vi "Autonomous Independent sensor.vi"() -> ()   [LabVIEW 2013]
doc: "This VI is called when autonomous begins, and will automatically be terminated when autonomous ends. You can carry out timed or sensor driven robot movement independently without needing to return to the caller."
uses:
  Robot Global Data.vi
  <vilib>/Rock Robotics/WPI/Joystick/WPI_JoystickGetSetRefNum.vi
  <vilib>/Rock Robotics/WPI/RobotDrive/WPI_RobotDriveGetSetRefNum.vi
  <vilib>/Rock Robotics/WPI/RobotDrive/WPI_RobotDriveArcadeDrive_Standard(NoSaturation).vi
panel:
  out "Auton Switch On?":bool
  out "Numeric 4":i32
  out "Numeric 3":i32
  out "Numeric 2":i32
  out "Numeric":i32
  out "distance (mm) 2":dbl
  out "Angle 2":dbl
  out "distance (mm)":dbl
  out "Current Movement, for debugging":T1 {"Y Joystick Value" scale=1.0..-1.0; "X Joystick Value" scale=-1.0..1.0}
  in  "Array of robot movements":T2(array[cluster]) {"Y Joystick Value" scale=1.0..-1.0; "X Joystick Value" scale=-1.0..1.0}
  # "Be sure to right-click and choose Data Operations>>Make Current Value default if you want to save the array values with the VI"
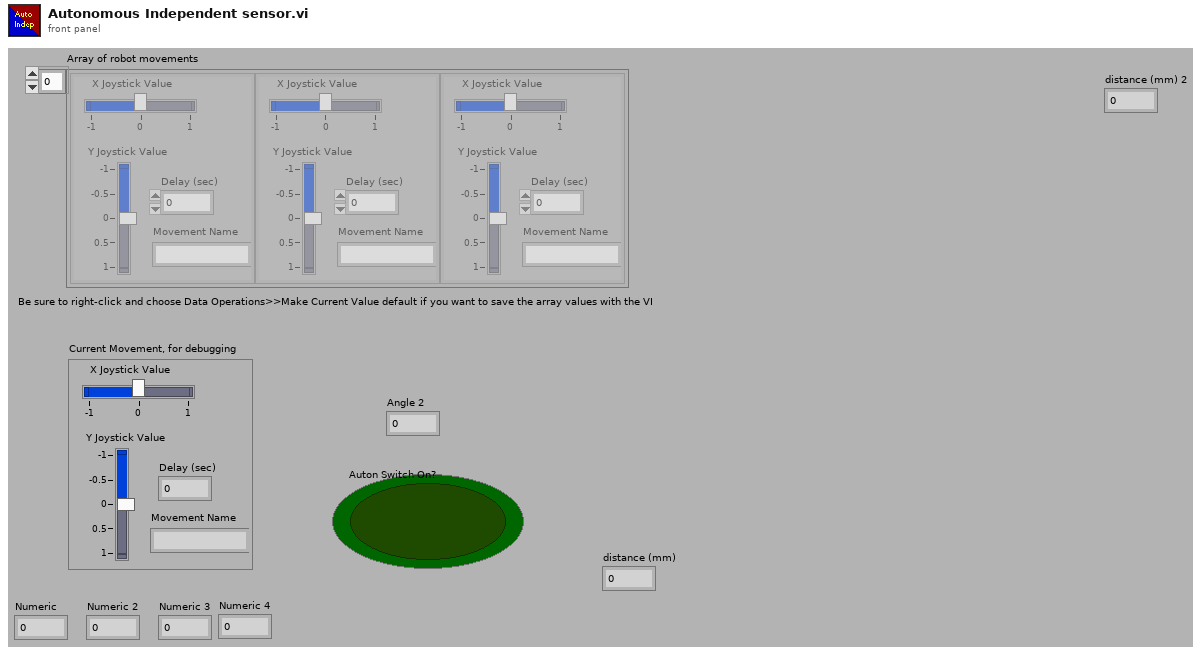
[diagram p1: front panel]
types:
  T1 = cluster{"X Joystick Value":dbl, "Y Joystick Value":dbl, "Delay (sec)":dbl, "Movement Name":string}
  T2 = cluster{"X Joystick Value":dbl, "Y Joystick Value":dbl, "Delay (sec)":dbl, "Movement Name":string}[]
  T3 = typedef "WPI_DigitalInputDevRef.ctl" = cluster{"DevStatus":errorcluster, "DIO Channel":T4, "Digital Module":T5}
  T4 = typedef "FPGA_DIOChannel.ctl" = enum8{"DIO 1", "DIO 2", "DIO 3", "DIO 4", "DIO 5", "DIO 6", "DIO 7", "DIO 8", "DIO 9", "DIO 10", "DIO 11", "DIO 12", "DIO 13", "DIO 14", "Invalid"}
  T5 = typedef "FPGA_TypedefDigitalModule.ctl" = enum16{"Digital Module 1", "Digital Module 2"}
  T6 = typedef "WPI_RobotDriveDevRef.ctl" = cluster{"DevStatus":errorcluster, "Motors[]":T7[], "Square Inputs":bool, "Max Output":dbl, "Isochronous":bool}
  T7 = typedef "WPI_MotorControlDeviceRef.ctl" = cluster{"DeviceStatus":errorcluster, "Type":enum16{"PWM", "CAN"}, "PWM":cluster{"Digital Module":T5, "PWM Channel":T8, "DeadBand":T9}, "CAN":cluster{"Device Number":u8, "Control Mode":T10, "Semaphore":T11, "Max Vout":dbl}, "Invert":bool, "TransformRef":T12, "InvTransformRef":T12}
  T8 = typedef "FPGA_DIOPWMChannel.ctl" = enum8{"PWM 1", "PWM 2", "PWM 3", "PWM 4", "PWM 5", "PWM 6", "PWM 7", "PWM 8", "PWM 9", "PWM 10", "Invalid"}
  T9 = typedef "WPI_PWMDeadband.ctl" = cluster{"Name":string, "maxPositivePwm":i32, "minPositivePwm":i32, "centerPwm":i32, "maxNegativePwm":i32, "minNegativePwm":i32, "angularRange":u16}
  T10 = typedef "WPI_CANJaguar_ControlMode.ctl" = enum8{"Percent VBus", "Current", "Speed", "Position", "Voltage"}
  T11 = typedef "Semaphore RefNum" = refnum<k1>
  T12 = typedef "WPI_PWMTransform_ConPane.ctl" = refnum<vi>
  T13 = typedef "WPI_GyroDevRef.ctl" = cluster{"DevStatus":errorcluster, "Analog Module":T14, "Analog Channel":T15, "Offset":dbl, "Gain (VoltsPerDegree/Second)":dbl}
  T14 = typedef "FPGA_TypedefAnalogModule.ctl" = enum16{"Analog Module 1", "Analog Module 2"}
  T15 = typedef "FPGA_AIChannel.ctl" = enum8{"AI 1", "AI 2", "AI 3", "AI 4", "AI 5", "AI 6", "AI 7", "AI 8", "Invalid"}
  T16 = typedef "WPI_AnalogChannelDevRef.ctl" = cluster{"DevStatus":errorcluster, "Analog Module":T14, "Analog Channel":T15}
  T17 = typedef "WPI_JoystickDevRef.ctl" = cluster{"Device":T18}
  T18 = typedef "WPI_JoystickDeviceEnum.ctl" = enum16{"USB 1", "USB 2", "USB 3", "USB 4", "Kinect 1", "Kinect 2"}
  T19 = cluster{"axis 1 (x)":dbl, "axis 2 (y)":dbl, "axis 3 (throttle)":dbl, "axis 4":dbl, "axis 5":dbl, "axis 6":dbl}
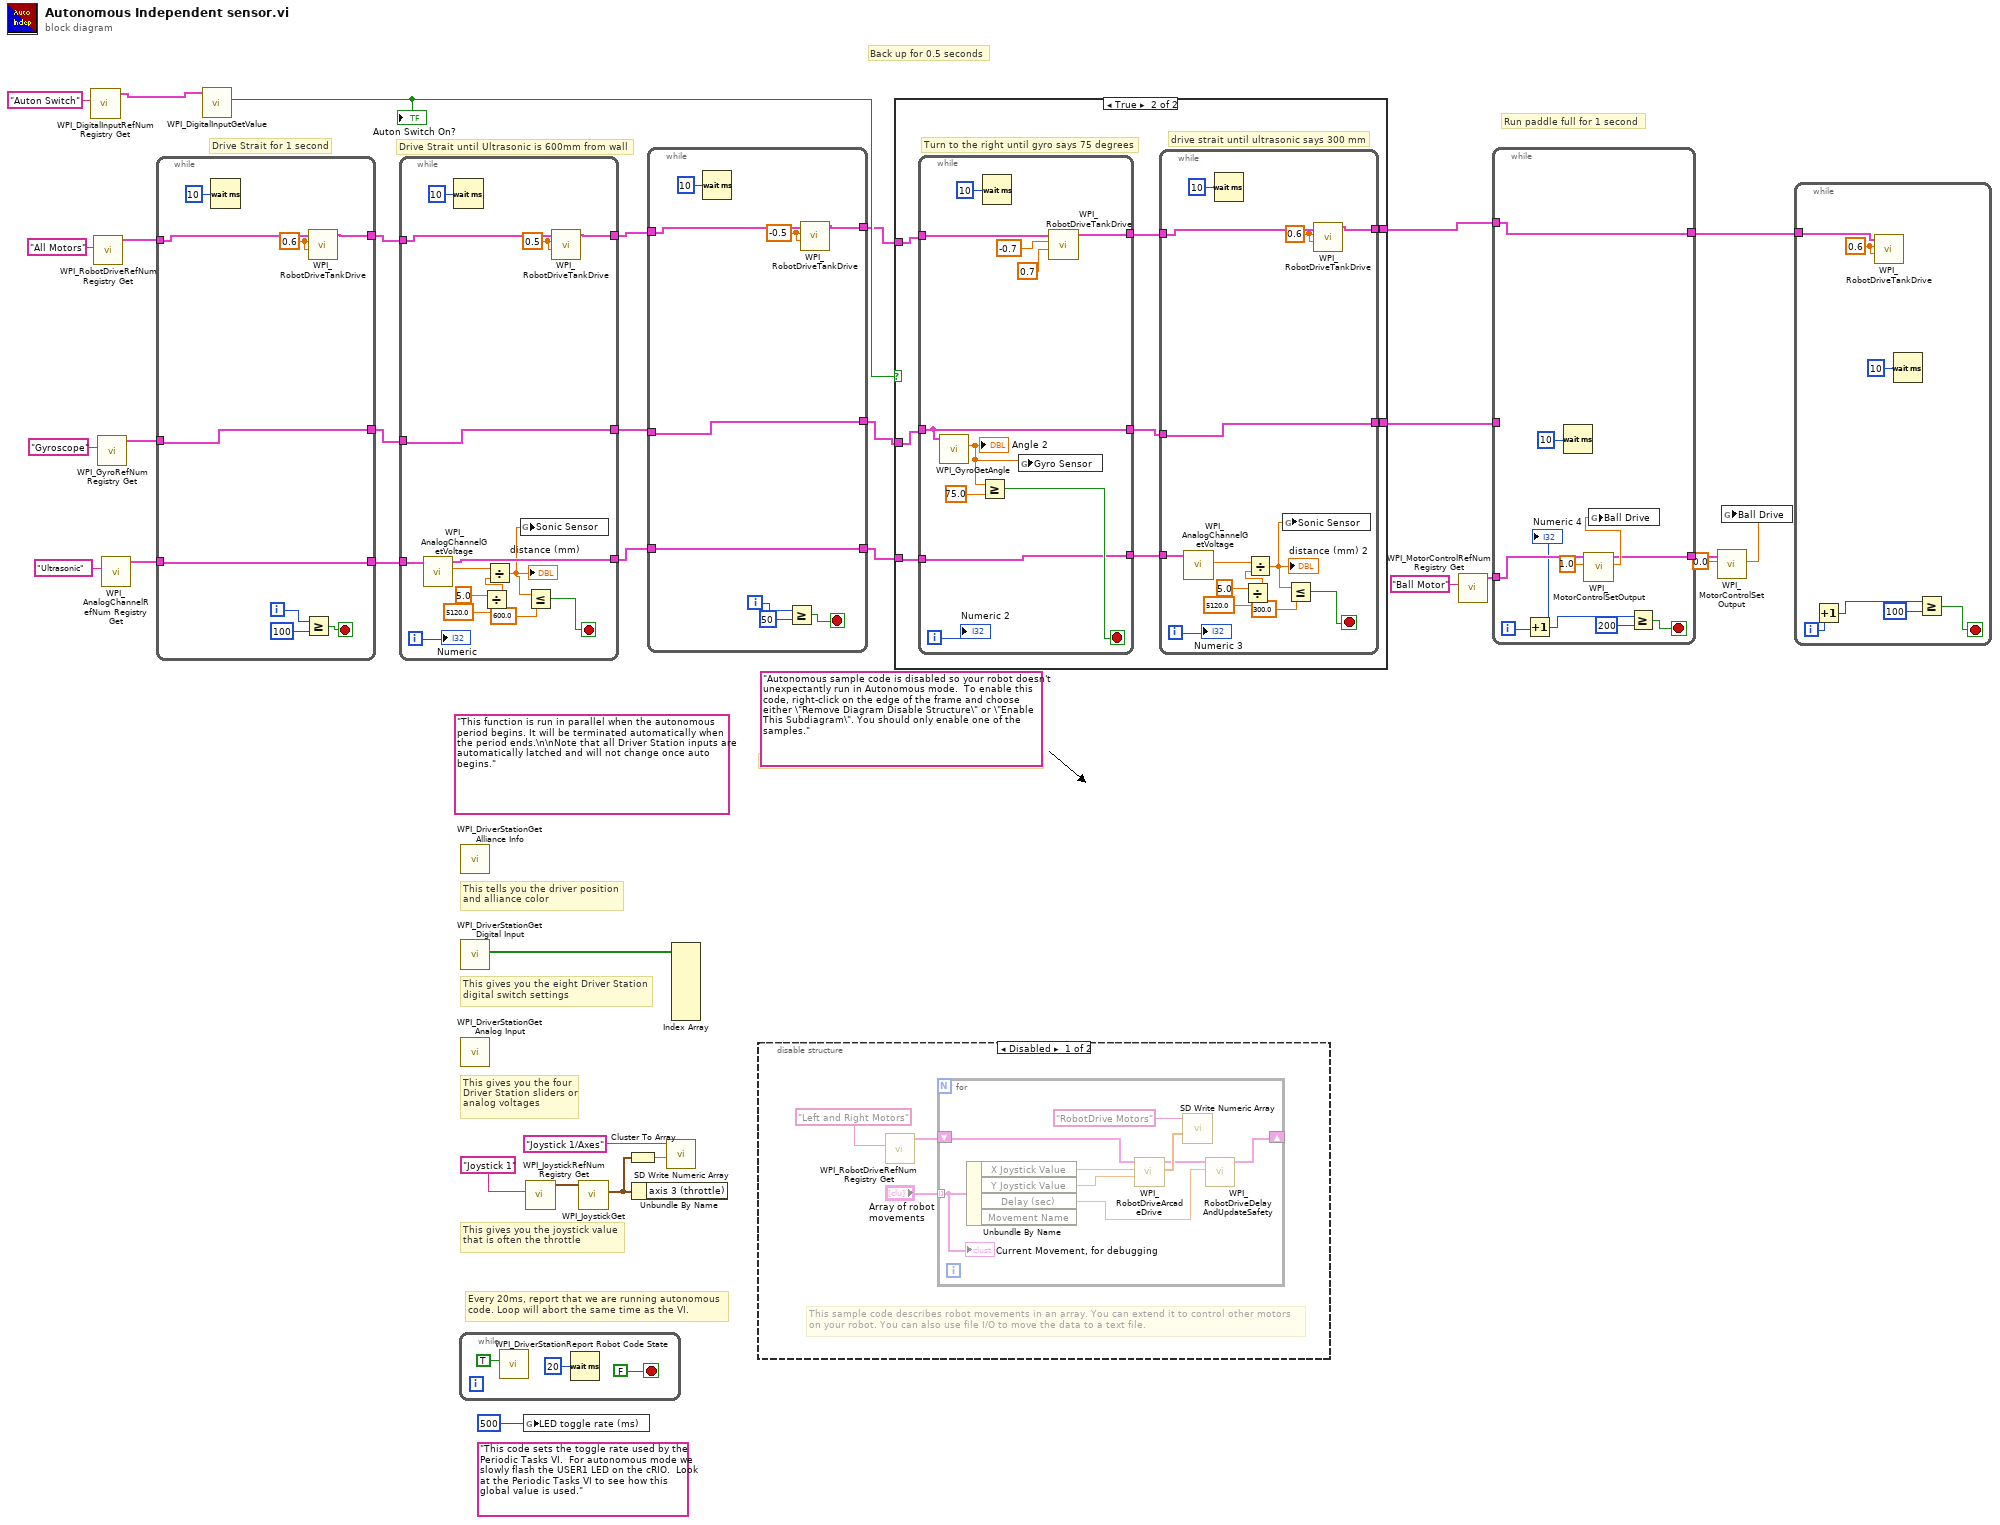
[diagram p0: block diagram]
diagram:
  (unwired) "This code sets the toggle rate used by the Periodic Tasks VI.  For autonomous mode we slowly flash the USER1 LED on the cRIO.  Look at the Periodic Tasks VI to see how this global value is used."
  (unwired) "Autonomous sample code is disabled so your robot doesn't unexpectantly run in Autonomous mode.  To enable this code, right-click on the edge of the frame and choose either \"Remove Diagram Disable Structure\" or \"Enable This Subdiagram\". You should only enable one of the samples."
  (unwired) "This function is run in parallel when the autonomous period begins. It will be terminated automatically when the period ends.\n\nNote that all Driver Station inputs are automatically latched and will not change once auto begins."
  # "Back up for 0.5 seconds"
  # "Run paddle full for 1 second"
  # "Drive Strait until Ultrasonic is 600mm from wall"
  # "Drive Strait for 1 second"
  # "Every 20ms, report that we are running autonomous\ncode. Loop will abort the same time as the VI."
  # "This gives you the joystick value\nthat is often the throttle"
  # "Use time and/or sensors to control how the robot drives."
  # "This tells you the driver position\nand alliance color"
  # "This gives you the eight Driver Station\ndigital switch settings"
  # "This gives you the four\nDriver Station sliders or\nanalog voltages"
  n1 = call <vilib>:"WPI_DigitalInputRefNum Registry Get.vi"("refnum name"="Auton Switch") -> ("DigitalInputDevRef"=w10:T3)  [unwired: 9 in, 1 out]
  n2 = call <vilib>:"WPI_RobotDriveRefNum Registry Get.vi"("refnum name"="All Motors") -> ("RobotDriveDevRef"=w16:T6)  [unwired: 9 in, 1 out]
  n3 = call <vilib>:"WPI_GyroRefNum Registry Get.vi"("refnum name"="Gyroscope") -> ("GyroDevRef"=w13:T13)  [unwired: 9 in, 1 out]
  n4 = call <vilib>:"WPI_AnalogChannelRefNum Registry Get.vi"("refnum name"="Ultrasonic") -> ("AIDeviceRef"=w17:T16)  [unwired: 9 in, 1 out]
  n5 = while {
    tunnel: w16 -> [w40]
    tunnel: w13 -> [w41]
    tunnel: [w39] -> w15
    tunnel: w17 -> [w37]
    tunnel: [w41] -> w12
    tunnel: [w37] -> w14
    i -> [w34]
    stop <- w35 stop-if-true
    w38 = 0.6 ("Left axis value")
    n6 = Wait (ms)(milliseconds to wait=u32 10) -> ()  [unwired: 1 out]
    n7 = Greater Or Equal?(x=w34, y=100) -> (x >= y?=w35:bool)
    n8 = call <vilib>:"WPI_RobotDriveTankDrive.vi"("Right axis value"=w38, "Left axis value"=w38, "RobotDriveDevRef"=w40) -> ("RobotDriveDevRef"=w39:T6)  [unwired: 6 in, 2 out]
  }
  n9 = call <vilib>:"WPI_DigitalInputGetValue.vi"("DigitalInputDevRef"=w10) -> ("Value"=w8:bool)  [unwired: 8 in, 2 out]
  "Auton Switch On?" <- w8
  n10 = while {
    tunnel: w15 -> [w45]
    tunnel: w12 -> [w46]
    tunnel: [w44] -> w7
    tunnel: w14 -> [w52]
    tunnel: [w46] -> w6
    tunnel: [w49] -> w5
    i -> [w47]
    stop <- w50 stop-if-true
    w43 = 0.5 ("Left axis value")
    n11 = call <vilib>:"WPI_AnalogChannelGetVoltage.vi"("AIDeviceRef"=w52) -> ("Voltage"=w55:dbl, "AIDeviceRef"=w49:T16)  [unwired: 8 in, 1 out]
    n12 = Wait (ms)(milliseconds to wait=u32 10) -> ()  [unwired: 1 out]
    n13 = Divide(x=5.0, y=5120.0) -> (x/y=w56:dbl)
    n14 = Divide(x=w55, y=w56) -> (x/y=w48:dbl)
    "distance (mm)" <- w48
    n15 = global write "Robot Global Data.vi" "Sonic Sensor"(w48) -> ()
    n16 = Less Or Equal?(x=w48, y=600.0) -> (x <= y?=w50:bool)
    n17 = call <vilib>:"WPI_RobotDriveTankDrive.vi"("Right axis value"=w43, "Left axis value"=w43, "RobotDriveDevRef"=w45) -> ("RobotDriveDevRef"=w44:T6)  [unwired: 6 in, 2 out]
    "Numeric" <- w47
  }
  n18 = while {
    stop <- FALSE stop-if-true
    n19 = call <vilib>:"WPI_DriverStationReport Robot Code State.vi"("Autonomous"=TRUE) -> ()  [unwired: 10 in, 1 out]
    n20 = Wait (ms)(milliseconds to wait=u32 20) -> ()  [unwired: 1 out]
  }
  n21 = call <vilib>:"WPI_DriverStationGet Alliance Info.vi"() -> ()  [unwired: 12 out]
  n22 = call <vilib>:"WPI_DriverStationGet Digital Input.vi"() -> ("Driver Station Digital Input (1-8)"=w33:bool[])  [unwired: 11 out]
  n23 = call <vilib>:"WPI_DriverStationGet Analog Input.vi"() -> ()  [unwired: 12 out]
  n24 = global write "Robot Global Data.vi" "LED toggle rate (ms)"(u32 500 ("LED ms toggle rate")) -> ()
  n25 = call <vilib>:"WPI_JoystickRefNum Registry Get.vi"("refnum name"="Joystick 1") -> ("JoystickDevRef"=w31:T17)  [unwired: 1 in, 9 out]
  n26 = call <vilib>:"WPI_JoystickGet.vi"("JoystickDevRef"=w31) -> ("Axes"=w28:T19)  [unwired: 1 in, 5 out]
  n27 = Cluster To Array(cluster=w28) -> (array=w29:dbl[])
  n28 = Unbundle By Name(w28) -> ()  [unwired: 1 out]
  n29 = while {
    tunnel: w7 -> [w67]
    tunnel: w6 -> [w68]
    tunnel: [w66] -> w4
    tunnel: [w68] -> w3
    tunnel: w5 -> [w64]
    tunnel: [w64] -> w2
    i -> [w63]
    stop <- w61 stop-if-true
    w65 = -0.5 ("Left axis value")
    n30 = Wait (ms)(milliseconds to wait=u32 10) -> ()  [unwired: 1 out]
    n31 = Greater Or Equal?(x=w63, y=50) -> (x >= y?=w61:bool)
    n32 = call <vilib>:"WPI_RobotDriveTankDrive.vi"("Right axis value"=w65, "Left axis value"=w65, "RobotDriveDevRef"=w67) -> ("RobotDriveDevRef"=w66:T6)  [unwired: 6 in, 2 out]
  }
  n33 = call <vilib>:"SD Write Numeric Array.vi"("Numeric Array"=w29, "Name"="Joystick 1/Axes") -> ()  [unwired: 8 in, 2 out]
  n34 = Index Array(array=w33) -> ()  [unwired: 8 in, 8 out]
  n35 = disable-structure shown="Disabled" {
    frame Disabled {
      # "This sample code describes robot movements in an array. You can extend it to control other motors\non your robot. You can also use file I/O to move the data to a text file."
      n36 = call <vilib>:"WPI_RobotDriveRefNum Registry Get.vi"("refnum name"="Left and Right Motors") -> ("RobotDriveDevRef"=w71:T6)  [unwired: 1 in, 9 out]
      n37 = for {
        shift-right: [w77] -> _
        shift-left: w71 -> [w78]
        tunnel: "Array of robot movements" -> [w73] mode=indexing
        n38 = Unbundle By Name(w73) -> ("X Joystick Value"=w76:dbl, "Y Joystick Value"=w75:dbl, "Delay (sec)"=w74:dbl)  [unwired: 1 out]
        n39 = call-poly <vilib>:"WPI_RobotDriveArcadeDrive.vi"("Y axis value"=w75, "X axis value"=w76, "RobotDriveDevRef"=w78) -> ("Motor Values"=w80:dbl[], "RobotDriveDevRef"=w79:T6)  [unwired: 1 in, 6 out]
        n40 = call <vilib>:"SD Write Numeric Array.vi"("Numeric Array"=w80, "Name"="RobotDrive Motors") -> ()  [unwired: 8 in, 2 out]
        n41 = call <vilib>:"WPI_RobotDriveDelayAndUpdateSafety.vi"("Delay (s)"=w74, "RobotDriveDevRef"=w79) -> ("RobotDriveDevRef 2"=w77:T6)  [unwired: 8 in, 1 out]
        "Current Movement, for debugging" <- w73
      }
    }
    frame Enabled {
    }
  }
  n42 = case shown="True" w8 {
    tunnel: [w83 w88] -> w22
    tunnel: w3 -> [w83 w86]
    tunnel: w4 -> [w82 w84]
    tunnel: [w82 w87] -> w9
    tunnel: w2 -> [_ w85]
    frame False {
    }
    frame True {
      # "drive strait until ultrasonic says 300 mm"
      # "Turn to the right until gyro says 75 degrees"
      n43 = while {
        tunnel: w84 -> [w109]
        tunnel: w86 -> [w113]
        tunnel: [w108] -> w91
        tunnel: [w113] -> w90
        tunnel: [w112] -> w89
        tunnel: w85 -> [w112]
        i -> [w110]
        stop <- w114 stop-if-true
        n44 = call <vilib>:"WPI_GyroGetAngle.vi"("GyroDevRef"=w113) -> ("Angle"=w111:dbl)  [unwired: 7 in, 3 out]
        "Angle 2" <- w111
        n45 = Greater Or Equal?(x=w111, y=75.0 ("setpoint")) -> (x >= y?=w114:bool)
        n46 = Wait (ms)(milliseconds to wait=u32 10) -> ()  [unwired: 1 out]
        n47 = global write "Robot Global Data.vi" "Gyro Sensor"(w111) -> ()
        n48 = call <vilib>:"WPI_RobotDriveTankDrive.vi"("Right axis value"=0.7, "Left axis value"=-0.7, "RobotDriveDevRef"=w109) -> ("RobotDriveDevRef"=w108:T6)  [unwired: 6 in, 2 out]
        "Numeric 2" <- w110
      }
      n49 = while {
        tunnel: w91 -> [w94]
        tunnel: w90 -> [w95]
        tunnel: [w93] -> w87
        tunnel: w89 -> [w100]
        tunnel: [w95] -> w88
        i -> [w96]
        stop <- w98 stop-if-true
        w92 = 0.6 ("Left axis value")
        n50 = call <vilib>:"WPI_AnalogChannelGetVoltage.vi"("AIDeviceRef"=w100) -> ("Voltage"=w103:dbl)  [unwired: 8 in, 2 out]
        n51 = Wait (ms)(milliseconds to wait=u32 10) -> ()  [unwired: 1 out]
        n52 = Divide(x=5.0, y=5120.0) -> (x/y=w104:dbl)
        n53 = Divide(x=w103, y=w104) -> (x/y=w97:dbl)
        "distance (mm) 2" <- w97
        n54 = global write "Robot Global Data.vi" "Sonic Sensor"(w97) -> ()
        n55 = Less Or Equal?(x=w97, y=300.0) -> (x <= y?=w98:bool)
        n56 = call <vilib>:"WPI_RobotDriveTankDrive.vi"("Right axis value"=w92, "Left axis value"=w92, "RobotDriveDevRef"=w94) -> ("RobotDriveDevRef"=w93:T6)  [unwired: 6 in, 2 out]
        "Numeric 3" <- w96
      }
    }
  }
  n57 = call <vilib>:"WPI_MotorControlRefNum Registry Get.vi"("refnum name"="Ball Motor") -> ("MotorControlDevRef"=w21:T7)  [unwired: 9 in, 1 out]
  n58 = while {
    tunnel: w22 -> [_]
    tunnel: w21 -> [w125]
    tunnel: [w118] -> w20
    tunnel: w9 -> [w117]
    tunnel: [w117] -> w1
    i -> [w123]
    stop <- w122 stop-if-true
    n59 = Increment(x=w123) -> (x+1=w121:i32)
    n60 = Wait (ms)(milliseconds to wait=u32 10) -> ()  [unwired: 1 out]
    n61 = call <vilib>:"WPI_MotorControlSetOutput.vi"("Output"=1.0, "MotorControlDevRef"=w125) -> ("Motor Output"=w119:dbl, "MotorControlDevRef"=w118:T7)  [unwired: 7 in, 1 out]
    n62 = global write "Robot Global Data.vi" "Ball Drive"(w119) -> ()
    n63 = Greater Or Equal?(x=w121, y=200) -> (x >= y?=w122:bool)
    "Numeric 4" <- w123
  }
  n64 = call <vilib>:"WPI_MotorControlSetOutput.vi"("Output"=0.0, "MotorControlDevRef"=w20) -> ("Motor Output"=w18:dbl)  [unwired: 7 in, 2 out]
  n65 = global write "Robot Global Data.vi" "Ball Drive"(w18) -> ()
  n66 = while {
    tunnel: w1 -> [w132]
    i -> [w128]
    stop <- w127 stop-if-true
    w133 = 0.6 ("Left axis value")
    n67 = Increment(x=w128) -> (x+1=w129:i32)
    n68 = call <vilib>:"WPI_RobotDriveTankDrive.vi"("Right axis value"=w133, "Left axis value"=w133, "RobotDriveDevRef"=w132) -> ()  [unwired: 6 in, 3 out]
    n69 = Wait (ms)(milliseconds to wait=u32 10) -> ()  [unwired: 1 out]
    n70 = Greater Or Equal?(x=w129, y=100) -> (x >= y?=w127:bool)
  }
